vi "Variant To Str.vi"(0 "data":variant, 11 "error in (no error)":errorcluster) -> (4 "JSON String":string, 15 "error out":errorcluster)   [LabVIEW 2019]
uses:
  <vilib>/addons/_JKI.lib/Serialization/JSON/JKI JSON Serialization.lvlib
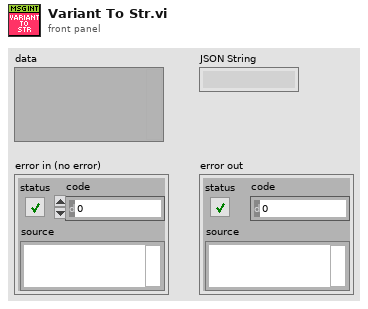
[diagram p1: front panel]
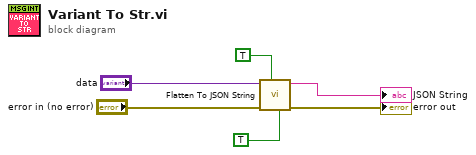
[diagram p0: block diagram]
diagram:
  n1 = call <vilib>:"Flatten To JSON String.vi"("Enums As String (F)"=TRUE, "Multiline (T)"=TRUE, "error in (no error)"="error in (no error)", "Variant"="data") -> ("error out"=→"error out":errorcluster, "JSON String"=→"JSON String":string)  [unwired: 6 in]
